vi "P9P14_Temp_Split_Cluster.vi"(0 "P9-P14 T-Cluster":T3 {"Temperature\nStatus" items=["TemperatureUnknown"=0, "Stable"=1, "Tracking"=2, "Near"=5, "Chasing"=6, "Filling"=7, "Standby"=10, "Disabled"=13, "ImpedanceNotFunction"=14, "TempFailure"=15]; "Approach" items=["Fast Settle", "No O'Shoot"]}) -> (1 "P9-P14 T-Cluster-Status":T1 {"Temperature\nStatus" items=["TemperatureUnknown"=0, "Stable"=1, "Tracking"=2, "Near"=5, "Chasing"=6, "Filling"=7, "Standby"=10, "Disabled"=13, "ImpedanceNotFunction"=14, "TempFailure"=15]}, 2 "P9-P14 T-Cluster -Control":T2 {"Approach" items=["Fast Settle", "No O'Shoot"]})   [LabVIEW 2019]
uses:
  PPMS/P9P14-TCluster.ctl
  PPMS/P9P14-TCluster-Control.ctl
  PPMS/P9P14-TCluster-Status.ctl
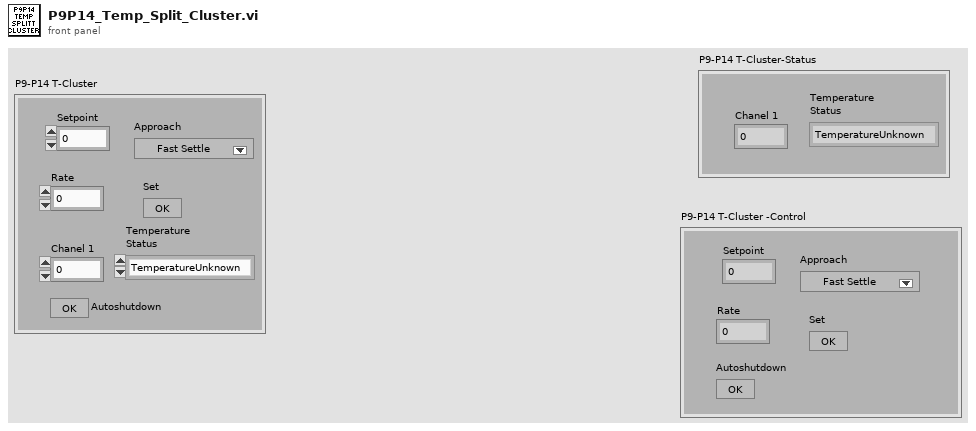
[diagram p1: front panel]
types:
  T1 = typedef "P9P14-TCluster-Status.ctl" = cluster{"Chanel 1":dbl, "Temperature\nStatus":i32}
  T2 = typedef "P9P14-TCluster-Control.ctl" = cluster{"Setpoint":dbl, "Rate":dbl, "Approach":u16, "Set":bool, "Autoshutdown":bool}
  T3 = typedef "P9P14-TCluster.ctl" = cluster{"Setpoint":dbl, "Rate":dbl, "Chanel 1":dbl, "Approach":u16, "Set":bool, "Temperature\nStatus":i32, "Autoshutdown":bool}
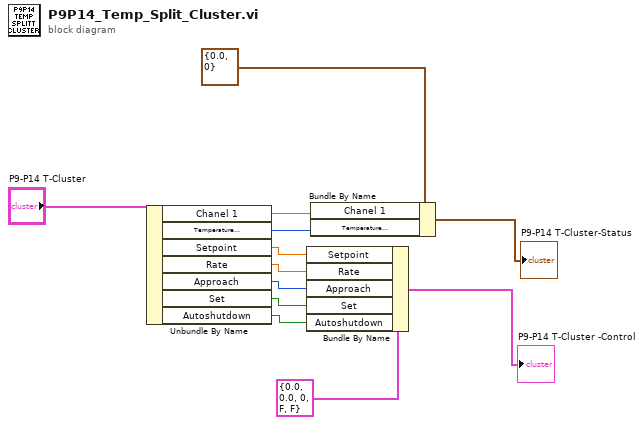
[diagram p0: block diagram]
diagram:
  n1 = Unbundle By Name("P9-P14 T-Cluster") -> ("Chanel 1"=w11:dbl, "Temperature\nStatus"=w10:i32, "Setpoint"=w5:dbl, "Rate"=w4:dbl, "Approach"=w3:u16, "Set"=w2:bool, "Autoshutdown"=w1:bool)
  n2 = Bundle By Name(cluster=T2 {"Setpoint"=0.0, "Rate"=0.0, "Approach"=0, "Set"=FALSE, "Autoshutdown"=FALSE} ("P9-P14 T-Cluster -Control 2"), "Setpoint"=w5, "Rate"=w4, "Approach"=w3, "Set"=w2, "Autoshutdown"=w1) -> (→"P9-P14 T-Cluster -Control":T2)
  n3 = Bundle By Name(cluster=T1 {"Chanel 1"=0.0, "Temperature\nStatus"=0} ("P9-P14 T-Cluster-Status 2"), "Chanel 1"=w11, "Temperature\nStatus"=w10) -> (→"P9-P14 T-Cluster-Status":T1)
